vi "dattotrace.vi"(2 "graph2list":u16, 3 "Current Average":sgl, 4 "graph1list":u16) -> (0 "trace2array out":sgl[](array[numeric]), 1 "trace1array out":sgl[](array[numeric]))   [LabVIEW 2015]
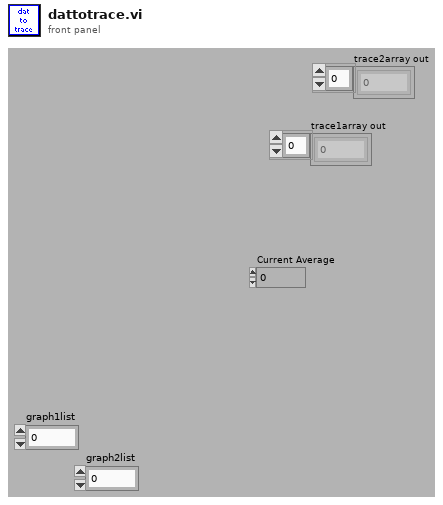
[diagram p1: front panel]
types:
  T1 = typedef "LVRectTypeDef.ctl" = cluster{"Left":i16, "Top":i16, "Right":i16, "Bottom":i16}
  T2 = cluster{"Xpixels":i32, "Vxminref":dbl, "Vxmaxref":dbl, "P":dbl, "Ypixels":i32, "Vyminref":dbl, "Vymaxref":dbl, "srate":sgl, "sAOxy":i32, "timeout":dbl, "type":string, "date":string, "time":string, "Colormap":u16, "Drawing Mode":u16, "Scanning Mode":u16, "square pixels":bool, "square matrix":bool, "Xpixels Img":i32, "Vx-min Img":dbl, "VX-max Img":dbl, "Ypixels Img":i32, "Vy-min Img":dbl, "Vy-max Img ":dbl, "Angle Img":dbl, "autoshutter":bool, "finite":bool, "cont":bool, "wavdet":bool, "measpoints":i32, "avpp":i32, "bufferAO":i32, "bufferAI":i32, "starttick":u32, "waveform":path, "Vx-ref":dbl, "Vy-ref":dbl, "refreshrate":dbl, "refreshbuffer":i32, "tt_cycles":i32, "motorref":refnum<k7>, "mirrorswitch":refnum<k7>, "sample mode":i32, "maxbufferAI":i32, "srateAODO":sgl, "bin":sgl, "Pel":sgl, "Angle draw":dbl, "srate Img":sgl, "ROIimg_plotbounds":T1, "auto OD":bool, "ODfilt":u16, "aAI":i32[], "aCI":i32[], "aAO":u32[], "aDO":u32[], "refwfsize":dbl, "Lifetime":bool, "Vz-Img":dbl, "Vz-ref":dbl, "Vz-reset":dbl, "AIoverride":bool, "aAS":u32[], "XYZstart":dbl[]}
  T3 = cluster{" AI":refnum<k21>, "E_AI":errorcluster, "header":dbl[]}
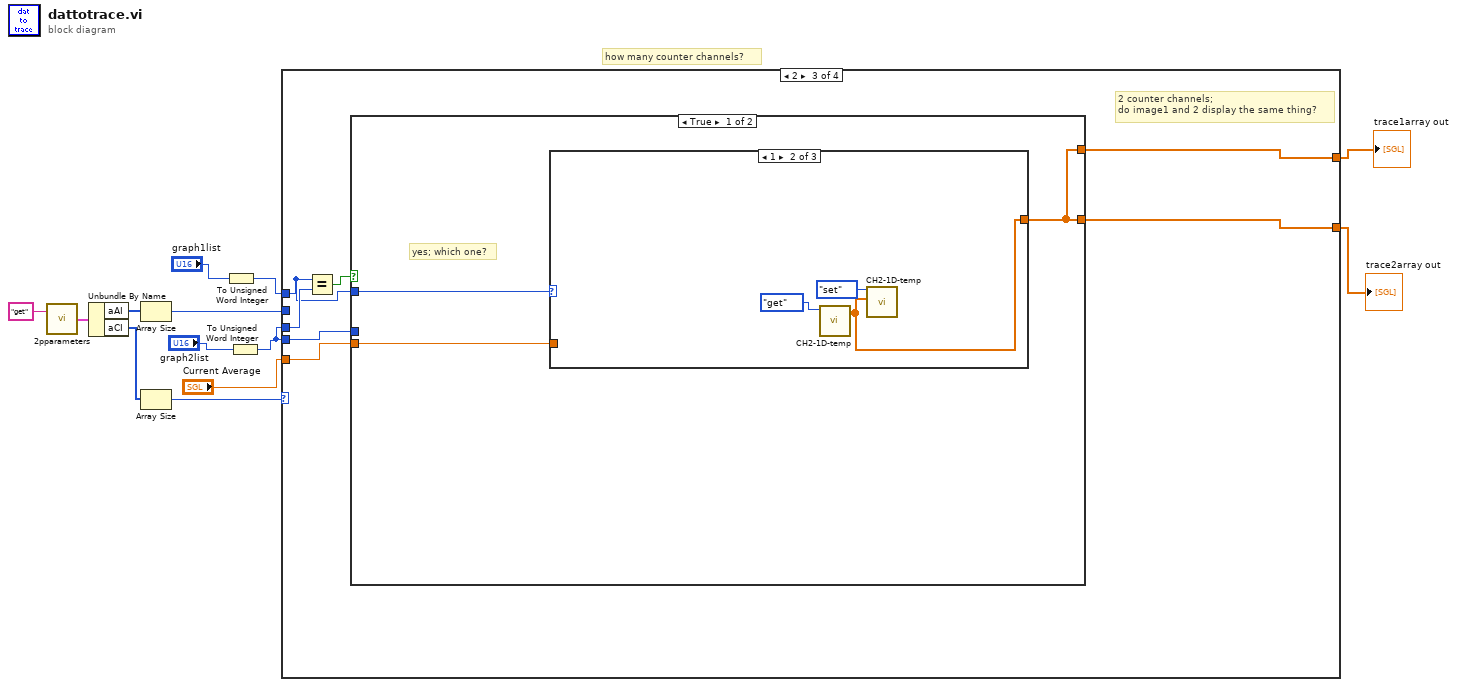
[diagram p0: block diagram]
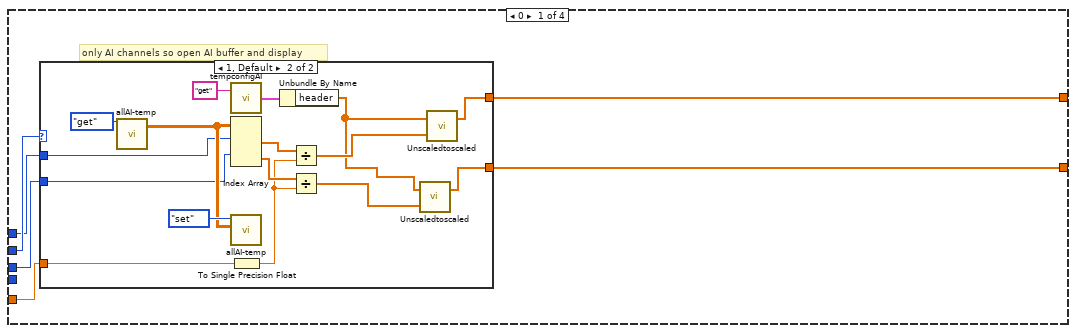
[diagram p2: hidden frame]
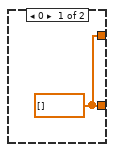
[diagram p3: hidden frame]
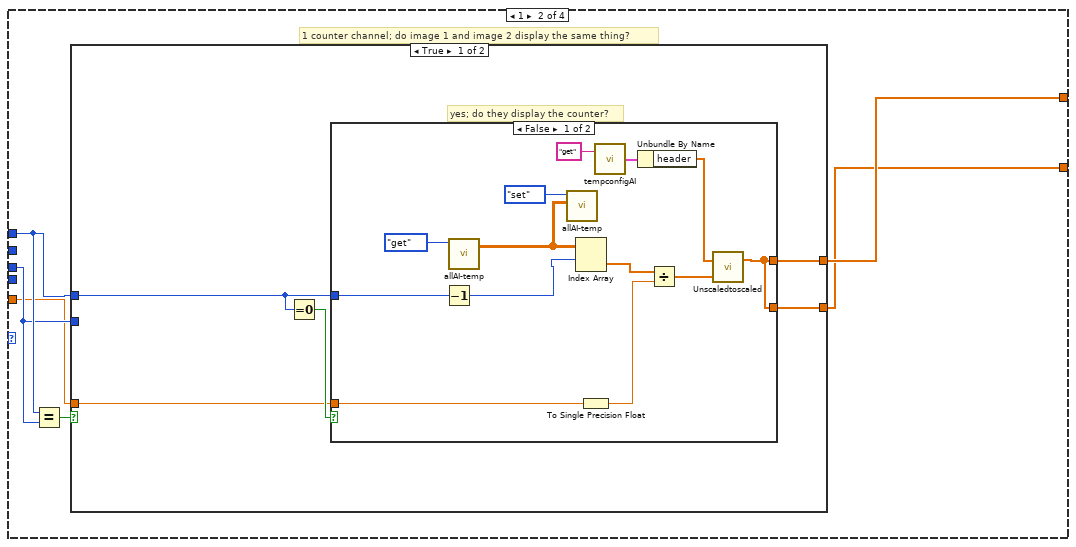
[diagram p4: hidden frame]
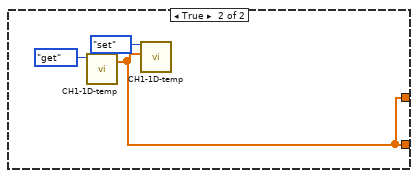
[diagram p5: hidden frame]
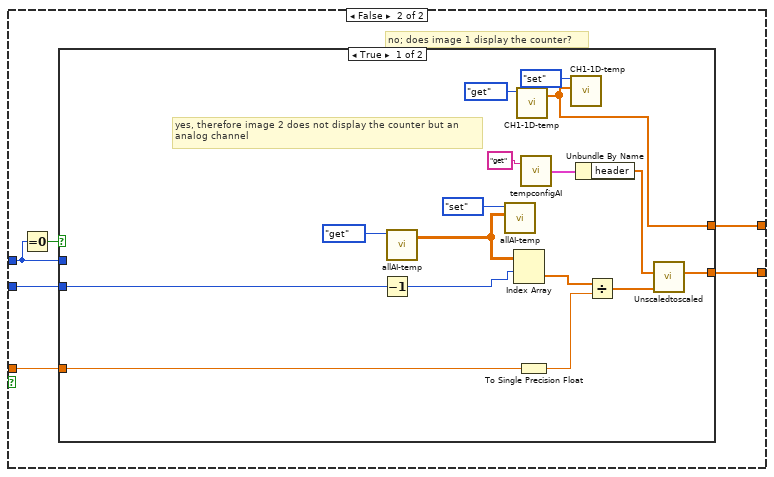
[diagram p6: hidden frame]
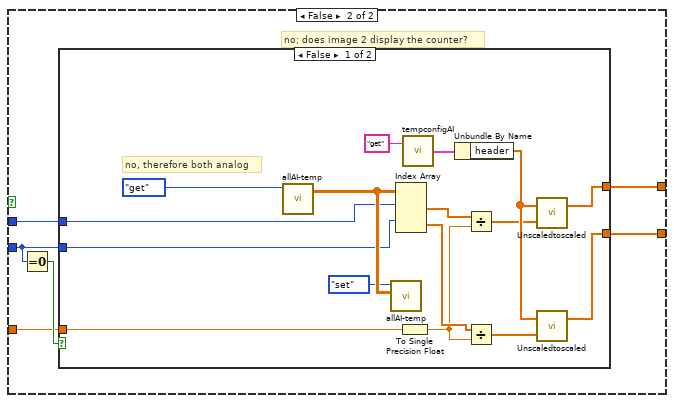
[diagram p7: hidden frame]
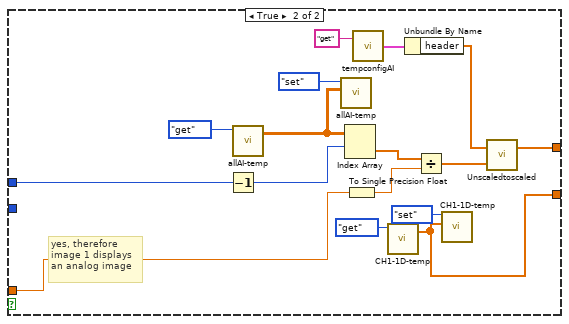
[diagram p8: hidden frame]
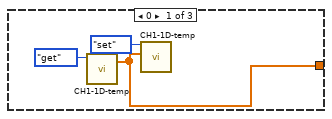
[diagram p9: hidden frame]
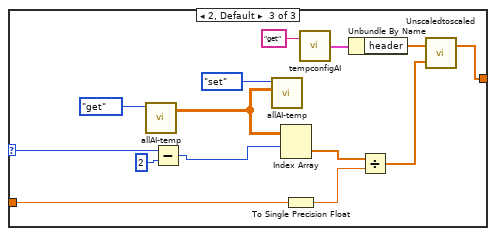
[diagram p10: hidden frame]
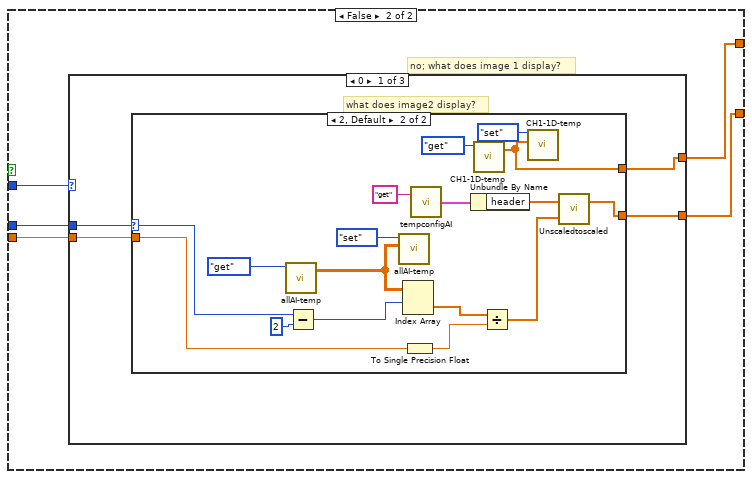
[diagram p11: hidden frame]
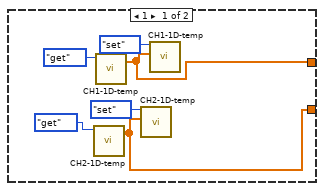
[diagram p12: hidden frame]
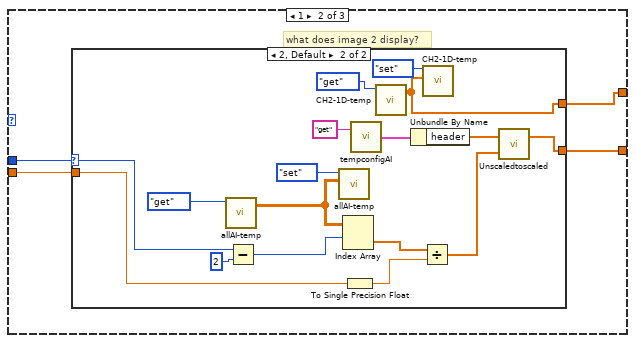
[diagram p13: hidden frame]
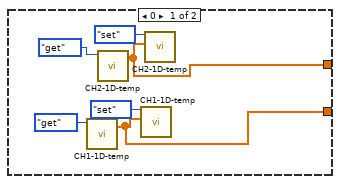
[diagram p14: hidden frame]
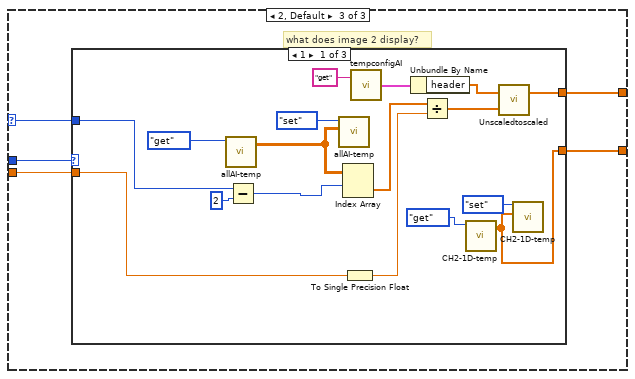
[diagram p15: hidden frame]
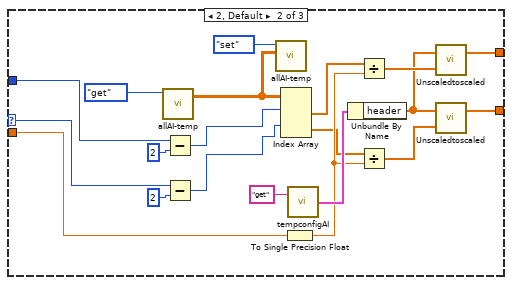
[diagram p16: hidden frame]
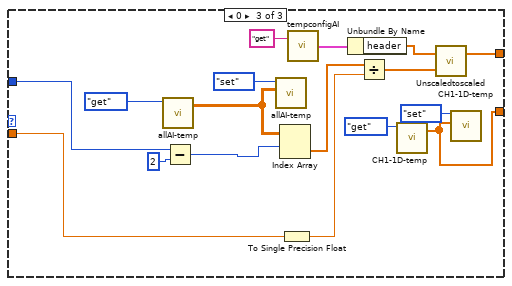
[diagram p17: hidden frame]
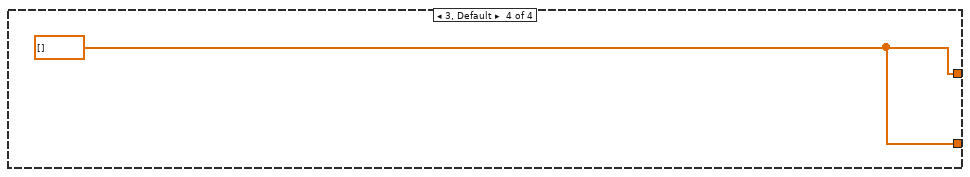
[diagram p18: hidden frame]
diagram:
  # "how many counter channels?"
  n1 = call "2pparameters.vi"("command"="get") -> ("params out"=w12:T2)  [unwired: 1 in]
  n2 = Unbundle By Name(w12) -> ("aAI"=w9:i32[], "aCI"=w11:i32[])
  n3 = Array Size(array=w9) -> (size(s)=w8:i32)
  n4 = Array Size(array=w11) -> (size(s)=w10:i32)
  n5 = To Unsigned Word Integer(number="graph1list") -> (unsigned 16bit integer=w4:u16)
  n6 = To Unsigned Word Integer(number="graph2list") -> (unsigned 16bit integer=w3:u16)
  n7 = case shown="2" w10 {
    tunnel: [w19 w42 w130 w272] -> w5
    tunnel: w8 -> [w18 _ _ _]
    tunnel: [w17 w39 w126 w272] -> w6
    tunnel: w4 -> [w16 w41 w127 _]
    tunnel: w3 -> [w15 w38 w129 _]
    tunnel: w3 -> [_ _ w125 _]
    tunnel: "Current Average" -> [w14 w37 w124 _]
    frame 0 {
      # "only AI channels so open AI buffer and display"
      n8 = case shown="1, Default" w18 {
        tunnel: [w20 w26] -> w19
        tunnel: [w20 w23] -> w17
        tunnel: w16 -> [_ w28]
        tunnel: w15 -> [_ w27]
        tunnel: w14 -> [_ w32]
        frame 0 {
          w20 = sgl[] []
        }
        frame 1, Default {
          n9 = call "allAI-temp.vi"("command"=enum16{"get", "set", "clear", "append"}."get") -> ("array out"=w29:sgl[][])  [unwired: 3 in, 1 out]
          n10 = call "tempconfigAI.vi"("command"="get") -> ("Temp Config out"=w35:T3)  [unwired: 1 in]
          n11 = Index Array(array=w29, index (row) #1=w28, index (row) #2=w27) -> (element #1=w33:sgl[], element #2=w22:sgl[])  [unwired: 2 in]
          n12 = call "allAI-temp.vi"("array in"=w29, "command"=enum16{"get", "set", "clear", "append"}."set") -> ()  [unwired: 2 in, 2 out]
          n13 = To Single Precision Float(number=w32) -> (single precision float=w21:sgl)
          n14 = Unbundle By Name(w35) -> ("header"=w25:dbl[])
          n15 = Divide(x=w33, y=w21) -> (x/y=w30:sgl[])
          n16 = Divide(x=w22, y=w21) -> (x/y=w24:sgl[])
          n17 = call "Unscaledtoscaled.vi"("Unscaled Data"=w24, "Header Information"=w25) -> ("Array"=w23:sgl[])  [unwired: 1 in]
          n18 = call "Unscaledtoscaled.vi"("Unscaled Data"=w30, "Header Information"=w25) -> ("Array"=w26:sgl[])  [unwired: 1 in]
        }
      }
    }
    frame 1 {
      # "1 counter channel; do image 1 and image 2 display the same thing?"
      n19 = Equal?(x=w41, y=w38) -> (x = y?=w40:bool)
      n20 = case shown="True" w40 {
        tunnel: [w47 w69] -> w42
        tunnel: w41 -> [w43 w65]
        tunnel: [w45 w67] -> w39
        tunnel: w38 -> [_ w66]
        tunnel: w37 -> [w44 w64]
        frame True {
          # "yes; do they display the counter?"
          n21 = Equal To 0?(x=w43) -> (x = 0?=w46:bool)
          n22 = case shown="False" w46 {
            tunnel: [w48 w61] -> w47
            tunnel: [w48 w61] -> w45
            tunnel: w44 -> [w53 _]
            tunnel: w43 -> [w52 _]
            frame False {
              n23 = Decrement(x=w52) -> (x-1=w51:u16)
              n24 = call "allAI-temp.vi"("command"=enum16{"get", "set", "clear", "append"}."get") -> ("array out"=w54:sgl[][])  [unwired: 3 in, 1 out]
              n25 = call "allAI-temp.vi"("array in"=w54, "command"=enum16{"get", "set", "clear", "append"}."set") -> ()  [unwired: 2 in, 2 out]
              n26 = Index Array(array=w54, index (row)=w51) -> (element=w56:sgl[])  [unwired: 1 in]
              n27 = To Single Precision Float(number=w53) -> (single precision float=w55:sgl)
              n28 = call "tempconfigAI.vi"("command"="get") -> ("Temp Config out"=w59:T3)  [unwired: 1 in]
              n29 = Unbundle By Name(w59) -> ("header"=w50:dbl[])
              n30 = Divide(x=w56, y=w55) -> (x/y=w49:sgl[])
              n31 = call "Unscaledtoscaled.vi"("Unscaled Data"=w49, "Header Information"=w50) -> ("Array"=w48:sgl[])  [unwired: 1 in]
            }
            frame True {
              n32 = call "CH1-1D-temp.vi"("command"=enum16{"get", "set", "clear", "append"}."get") -> ("array out"=w61:sgl[])  [unwired: 3 in, 1 out]
              n33 = call "CH1-1D-temp.vi"("array in"=w61, "command"=enum16{"get", "set", "clear", "append"}."set") -> ()  [unwired: 2 in, 2 out]
            }
          }
        }
        frame False {
          # "no; does image 1 display the counter?"
          n34 = Equal To 0?(x=w65) -> (x = 0?=w68:bool)
          n35 = case shown="True" w68 {
            tunnel: [w74 w90] -> w69
            tunnel: [w70 w89] -> w67
            tunnel: w66 -> [w79 w87]
            tunnel: w65 -> [_ w91]
            tunnel: w64 -> [w77 w86]
            frame True {
              # "yes, therefore image 2 does not display the counter but an\nanalog channel"
              n36 = Decrement(x=w79) -> (x-1=w73:u16)
              n37 = call "allAI-temp.vi"("command"=enum16{"get", "set", "clear", "append"}."get") -> ("array out"=w78:sgl[][])  [unwired: 3 in, 1 out]
              n38 = call "allAI-temp.vi"("array in"=w78, "command"=enum16{"get", "set", "clear", "append"}."set") -> ()  [unwired: 2 in, 2 out]
              n39 = Index Array(array=w78, index (row)=w73) -> (element=w81:sgl[])  [unwired: 1 in]
              n40 = call "CH1-1D-temp.vi"("command"=enum16{"get", "set", "clear", "append"}."get") -> ("array out"=w74:sgl[])  [unwired: 3 in, 1 out]
              n41 = To Single Precision Float(number=w77) -> (single precision float=w80:sgl)
              n42 = call "tempconfigAI.vi"("command"="get") -> ("Temp Config out"=w84:T3)  [unwired: 1 in]
              n43 = call "CH1-1D-temp.vi"("array in"=w74, "command"=enum16{"get", "set", "clear", "append"}."set") -> ()  [unwired: 2 in, 2 out]
              n44 = Unbundle By Name(w84) -> ("header"=w72:dbl[])
              n45 = Divide(x=w81, y=w80) -> (x/y=w71:sgl[])
              n46 = call "Unscaledtoscaled.vi"("Unscaled Data"=w71, "Header Information"=w72) -> ("Array"=w70:sgl[])  [unwired: 1 in]
            }
            frame False {
              # "no; does image 2 display the counter?"
              n47 = Equal To 0?(x=w87) -> (x = 0?=w88:bool)
              n48 = case shown="False" w88 {
                tunnel: w91 -> [w95 w114]
                tunnel: [w97 w113] -> w90
                tunnel: [w98 w108] -> w89
                tunnel: w87 -> [w94 _]
                tunnel: w86 -> [w96 w112]
                frame False {
                  # "no, therefore both analog"
                  n49 = call "allAI-temp.vi"("command"=enum16{"get", "set", "clear", "append"}."get") -> ("array out"=w104:sgl[][])  [unwired: 3 in, 1 out]
                  n50 = call "allAI-temp.vi"("array in"=w104, "command"=enum16{"get", "set", "clear", "append"}."set") -> ()  [unwired: 2 in, 2 out]
                  n51 = Index Array(array=w104, index (row) #1=w95, index (row) #2=w94) -> (element #1=w103:sgl[], element #2=w93:sgl[])  [unwired: 2 in]
                  n52 = To Single Precision Float(number=w96) -> (single precision float=w92:sgl)
                  n53 = call "tempconfigAI.vi"("command"="get") -> ("Temp Config out"=w100:T3)  [unwired: 1 in]
                  n54 = Unbundle By Name(w100) -> ("header"=w106:dbl[])
                  n55 = Divide(x=w103, y=w92) -> (x/y=w105:sgl[])
                  n56 = Divide(x=w93, y=w92) -> (x/y=w107:sgl[])
                  n57 = call "Unscaledtoscaled.vi"("Unscaled Data"=w105, "Header Information"=w106) -> ("Array"=w97:sgl[])  [unwired: 1 in]
                  n58 = call "Unscaledtoscaled.vi"("Unscaled Data"=w107, "Header Information"=w106) -> ("Array"=w98:sgl[])  [unwired: 1 in]
                }
                frame True {
                  # "yes, therefore\nimage 1 displays \nan analog image"
                  n59 = Decrement(x=w114) -> (x-1=w111:u16)
                  n60 = call "allAI-temp.vi"("command"=enum16{"get", "set", "clear", "append"}."get") -> ("array out"=w115:sgl[][])  [unwired: 3 in, 1 out]
                  n61 = call "allAI-temp.vi"("array in"=w115, "command"=enum16{"get", "set", "clear", "append"}."set") -> ()  [unwired: 2 in, 2 out]
                  n62 = Index Array(array=w115, index (row)=w111) -> (element=w118:sgl[])  [unwired: 1 in]
                  n63 = To Single Precision Float(number=w112) -> (single precision float=w117:sgl)
                  n64 = call "tempconfigAI.vi"("command"="get") -> ("Temp Config out"=w122:T3)  [unwired: 1 in]
                  n65 = call "CH1-1D-temp.vi"("command"=enum16{"get", "set", "clear", "append"}."get") -> ("array out"=w108:sgl[])  [unwired: 3 in, 1 out]
                  n66 = Unbundle By Name(w122) -> ("header"=w121:dbl[])
                  n67 = Divide(x=w118, y=w117) -> (x/y=w116:sgl[])
                  n68 = call "CH1-1D-temp.vi"("array in"=w108, "command"=enum16{"get", "set", "clear", "append"}."set") -> ()  [unwired: 2 in, 2 out]
                  n69 = call "Unscaledtoscaled.vi"("Unscaled Data"=w116, "Header Information"=w121) -> ("Array"=w113:sgl[])  [unwired: 1 in]
                }
              }
            }
          }
        }
      }
    }
    frame 2 {
      # "2 counter channels;\ndo image1 and 2 display the same thing?"
      n70 = Equal?(x=w127, y=w129) -> (x = y?=w128:bool)
      n71 = case shown="True" w128 {
        tunnel: [w133 w157] -> w130
        tunnel: w127 -> [w131 w158]
        tunnel: [w133 w155] -> w126
        tunnel: w125 -> [_ w156]
        tunnel: w124 -> [w132 w154]
        frame True {
          # "yes; which one?"
          n72 = case shown="1" w131 {
            selector: w131 -> [_ _ w142]
            tunnel: [w134 w137 w144] -> w133
            tunnel: w132 -> [_ _ w141]
            frame 0 {
              n73 = call "CH1-1D-temp.vi"("command"=enum16{"get", "set", "clear", "append"}."get") -> ("array out"=w134:sgl[])  [unwired: 3 in, 1 out]
              n74 = call "CH1-1D-temp.vi"("array in"=w134, "command"=enum16{"get", "set", "clear", "append"}."set") -> ()  [unwired: 2 in, 2 out]
            }
            frame 1 {
              n75 = call "CH2-1D-temp.vi"("command"=enum16{"get", "set", "clear", "append"}."get") -> ("array out"=w137:sgl[])  [unwired: 3 in, 1 out]
              n76 = call "CH2-1D-temp.vi"("array in"=w137, "command"=enum16{"get", "set", "clear", "append"}."set") -> ()  [unwired: 2 in, 2 out]
            }
            frame 2, Default {
              n77 = call "allAI-temp.vi"("command"=enum16{"get", "set", "clear", "append"}."get") -> ("array out"=w146:sgl[][])  [unwired: 3 in, 1 out]
              n78 = Subtract(x=w142, y=2) -> (x-y=w140:i32)
              n79 = call "allAI-temp.vi"("array in"=w146, "command"=enum16{"get", "set", "clear", "append"}."set") -> ()  [unwired: 2 in, 2 out]
              n80 = Index Array(array=w146, index (row)=w140) -> (element=w148:sgl[])  [unwired: 1 in]
              n81 = To Single Precision Float(number=w141) -> (single precision float=w147:sgl)
              n82 = call "tempconfigAI.vi"("command"="get") -> ("Temp Config out"=w152:T3)  [unwired: 1 in]
              n83 = Unbundle By Name(w152) -> ("header"=w151:dbl[])
              n84 = Divide(x=w148, y=w147) -> (x/y=w145:sgl[])
              n85 = call "Unscaledtoscaled.vi"("Unscaled Data"=w145, "Header Information"=w151) -> ("Array"=w144:sgl[])  [unwired: 1 in]
            }
          }
        }
        frame False {
          # "no; what does image 1 display?"
          n86 = case shown="0" w158 {
            selector: w158 -> [_ _ w216]
            tunnel: [w162 w189 w217] -> w157
            tunnel: w156 -> [w161 w188 w215]
            tunnel: [w160 w187 w214] -> w155
            tunnel: w154 -> [w159 w186 w213]
            frame 0 {
              # "what does image2 display?"
              n87 = case shown="2, Default" w161 {
                selector: w161 -> [_ w175]
                tunnel: [w166 w170] -> w162
                tunnel: [w163 w174] -> w160
                tunnel: w159 -> [_ w173]
                frame 1 {
                  n88 = call "CH2-1D-temp.vi"("command"=enum16{"get", "set", "clear", "append"}."get") -> ("array out"=w163:sgl[])  [unwired: 3 in, 1 out]
                  n89 = call "CH1-1D-temp.vi"("command"=enum16{"get", "set", "clear", "append"}."get") -> ("array out"=w166:sgl[])  [unwired: 3 in, 1 out]
                  n90 = call "CH2-1D-temp.vi"("array in"=w163, "command"=enum16{"get", "set", "clear", "append"}."set") -> ()  [unwired: 2 in, 2 out]
                  n91 = call "CH1-1D-temp.vi"("array in"=w166, "command"=enum16{"get", "set", "clear", "append"}."set") -> ()  [unwired: 2 in, 2 out]
                }
                frame 2, Default {
                  n92 = call "allAI-temp.vi"("command"=enum16{"get", "set", "clear", "append"}."get") -> ("array out"=w178:sgl[][])  [unwired: 3 in, 1 out]
                  n93 = Subtract(x=w175, y=2) -> (x-y=w169:i32)
                  n94 = call "allAI-temp.vi"("array in"=w178, "command"=enum16{"get", "set", "clear", "append"}."set") -> ()  [unwired: 2 in, 2 out]
                  n95 = Index Array(array=w178, index (row)=w169) -> (element=w180:sgl[])  [unwired: 1 in]
                  n96 = To Single Precision Float(number=w173) -> (single precision float=w179:sgl)
                  n97 = call "tempconfigAI.vi"("command"="get") -> ("Temp Config out"=w184:T3)  [unwired: 1 in]
                  n98 = Unbundle By Name(w184) -> ("header"=w183:dbl[])
                  n99 = call "CH1-1D-temp.vi"("command"=enum16{"get", "set", "clear", "append"}."get") -> ("array out"=w170:sgl[])  [unwired: 3 in, 1 out]
                  n100 = Divide(x=w180, y=w179) -> (x/y=w177:sgl[])
                  n101 = call "CH1-1D-temp.vi"("array in"=w170, "command"=enum16{"get", "set", "clear", "append"}."set") -> ()  [unwired: 2 in, 2 out]
                  n102 = call "Unscaledtoscaled.vi"("Unscaled Data"=w177, "Header Information"=w183) -> ("Array"=w174:sgl[])  [unwired: 1 in]
                }
              }
            }
            frame 1 {
              # "what does image 2 display?"
              n103 = case shown="2, Default" w188 {
                selector: w188 -> [_ w202]
                tunnel: [w193 w197] -> w189
                tunnel: [w190 w201] -> w187
                tunnel: w186 -> [_ w200]
                frame 0 {
                  n104 = call "CH1-1D-temp.vi"("command"=enum16{"get", "set", "clear", "append"}."get") -> ("array out"=w190:sgl[])  [unwired: 3 in, 1 out]
                  n105 = call "CH2-1D-temp.vi"("command"=enum16{"get", "set", "clear", "append"}."get") -> ("array out"=w193:sgl[])  [unwired: 3 in, 1 out]
                  n106 = call "CH1-1D-temp.vi"("array in"=w190, "command"=enum16{"get", "set", "clear", "append"}."set") -> ()  [unwired: 2 in, 2 out]
                  n107 = call "CH2-1D-temp.vi"("array in"=w193, "command"=enum16{"get", "set", "clear", "append"}."set") -> ()  [unwired: 2 in, 2 out]
                }
                frame 2, Default {
                  n108 = call "allAI-temp.vi"("command"=enum16{"get", "set", "clear", "append"}."get") -> ("array out"=w205:sgl[][])  [unwired: 3 in, 1 out]
                  n109 = Subtract(x=w202, y=2) -> (x-y=w196:i32)
                  n110 = call "allAI-temp.vi"("array in"=w205, "command"=enum16{"get", "set", "clear", "append"}."set") -> ()  [unwired: 2 in, 2 out]
                  n111 = Index Array(array=w205, index (row)=w196) -> (element=w207:sgl[])  [unwired: 1 in]
                  n112 = To Single Precision Float(number=w200) -> (single precision float=w206:sgl)
                  n113 = call "tempconfigAI.vi"("command"="get") -> ("Temp Config out"=w211:T3)  [unwired: 1 in]
                  n114 = call "CH2-1D-temp.vi"("command"=enum16{"get", "set", "clear", "append"}."get") -> ("array out"=w197:sgl[])  [unwired: 3 in, 1 out]
                  n115 = Unbundle By Name(w211) -> ("header"=w210:dbl[])
                  n116 = Divide(x=w207, y=w206) -> (x/y=w204:sgl[])
                  n117 = call "CH2-1D-temp.vi"("array in"=w197, "command"=enum16{"get", "set", "clear", "append"}."set") -> ()  [unwired: 2 in, 2 out]
                  n118 = call "Unscaledtoscaled.vi"("Unscaled Data"=w204, "Header Information"=w210) -> ("Array"=w201:sgl[])  [unwired: 1 in]
                }
              }
            }
            frame 2, Default {
              # "what does image 2 display?"
              n119 = case shown="1" w215 {
                selector: w215 -> [_ w243 _]
                tunnel: [w225 w247 w262] -> w217
                tunnel: w216 -> [w223 w245 w260]
                tunnel: [w218 w238 w256] -> w214
                tunnel: w213 -> [w222 w237 w259]
                frame 1 {
                  n120 = call "allAI-temp.vi"("command"=enum16{"get", "set", "clear", "append"}."get") -> ("array out"=w227:sgl[][])  [unwired: 3 in, 1 out]
                  n121 = Subtract(x=w223, y=2) -> (x-y=w221:i32)
                  n122 = call "allAI-temp.vi"("array in"=w227, "command"=enum16{"get", "set", "clear", "append"}."set") -> ()  [unwired: 2 in, 2 out]
                  n123 = Index Array(array=w227, index (row)=w221) -> (element=w229:sgl[])  [unwired: 1 in]
                  n124 = To Single Precision Float(number=w222) -> (single precision float=w228:sgl)
                  n125 = call "tempconfigAI.vi"("command"="get") -> ("Temp Config out"=w233:T3)  [unwired: 1 in]
                  n126 = Unbundle By Name(w233) -> ("header"=w232:dbl[])
                  n127 = Divide(x=w229, y=w228) -> (x/y=w226:sgl[])
                  n128 = call "CH2-1D-temp.vi"("command"=enum16{"get", "set", "clear", "append"}."get") -> ("array out"=w218:sgl[])  [unwired: 3 in, 1 out]
                  n129 = call "Unscaledtoscaled.vi"("Unscaled Data"=w226, "Header Information"=w232) -> ("Array"=w225:sgl[])  [unwired: 1 in]
                  n130 = call "CH2-1D-temp.vi"("array in"=w218, "command"=enum16{"get", "set", "clear", "append"}."set") -> ()  [unwired: 2 in, 2 out]
                }
                frame 2, Default {
                  n131 = call "allAI-temp.vi"("command"=enum16{"get", "set", "clear", "append"}."get") -> ("array out"=w249:sgl[][])  [unwired: 3 in, 1 out]
                  n132 = Subtract(x=w245, y=2) -> (x-y=w235:i32)
                  n133 = Subtract(x=w243, y=2) -> (x-y=w236:i32)
                  n134 = call "allAI-temp.vi"("array in"=w249, "command"=enum16{"get", "set", "clear", "append"}."set") -> ()  [unwired: 2 in, 2 out]
                  n135 = Index Array(array=w249, index (row) #1=w235, index (row) #2=w236) -> (element #1=w250:sgl[], element #2=w241:sgl[])  [unwired: 2 in]
                  n136 = To Single Precision Float(number=w237) -> (single precision float=w242:sgl)
                  n137 = call "tempconfigAI.vi"("command"="get") -> ("Temp Config out"=w253:T3)  [unwired: 1 in]
                  n138 = Unbundle By Name(w253) -> ("header"=w240:dbl[])
                  n139 = Divide(x=w250, y=w242) -> (x/y=w248:sgl[])
                  n140 = Divide(x=w241, y=w242) -> (x/y=w239:sgl[])
                  n141 = call "Unscaledtoscaled.vi"("Unscaled Data"=w248, "Header Information"=w240) -> ("Array"=w247:sgl[])  [unwired: 1 in]
                  n142 = call "Unscaledtoscaled.vi"("Unscaled Data"=w239, "Header Information"=w240) -> ("Array"=w238:sgl[])  [unwired: 1 in]
                }
                frame 0 {
                  n143 = call "allAI-temp.vi"("command"=enum16{"get", "set", "clear", "append"}."get") -> ("array out"=w264:sgl[][])  [unwired: 3 in, 1 out]
                  n144 = Subtract(x=w260, y=2) -> (x-y=w255:i32)
                  n145 = call "allAI-temp.vi"("array in"=w264, "command"=enum16{"get", "set", "clear", "append"}."set") -> ()  [unwired: 2 in, 2 out]
                  n146 = Index Array(array=w264, index (row)=w255) -> (element=w266:sgl[])  [unwired: 1 in]
                  n147 = To Single Precision Float(number=w259) -> (single precision float=w265:sgl)
                  n148 = call "tempconfigAI.vi"("command"="get") -> ("Temp Config out"=w270:T3)  [unwired: 1 in]
                  n149 = Unbundle By Name(w270) -> ("header"=w269:dbl[])
                  n150 = Divide(x=w266, y=w265) -> (x/y=w263:sgl[])
                  n151 = call "CH1-1D-temp.vi"("command"=enum16{"get", "set", "clear", "append"}."get") -> ("array out"=w256:sgl[])  [unwired: 3 in, 1 out]
                  n152 = call "Unscaledtoscaled.vi"("Unscaled Data"=w263, "Header Information"=w269) -> ("Array"=w262:sgl[])  [unwired: 1 in]
                  n153 = call "CH1-1D-temp.vi"("array in"=w256, "command"=enum16{"get", "set", "clear", "append"}."set") -> ()  [unwired: 2 in, 2 out]
                }
              }
            }
          }
        }
      }
    }
    frame 3, Default {
      w272 = sgl[] []
    }
  }
  "trace1array out" <- w5
  "trace2array out" <- w6
